vi "Home.vi"(7 "error in (no error)":errorcluster caption="에러 입력(에러 없음)") -> (0 "error out":errorcluster caption="에러 출력", 2 "State":T1)   [LabVIEW 2019]
uses:
  controller/patientListBtn.ctl
  controller/robotBtn.ctl
  controller/alignBtn.ctl
  controller/exitBtn.ctl
  controller/logoutBtn.ctl
  controller/pannelState.ctl
  <vilib>/Utility/miscctls.llb/LVPointTypeDef.ctl
  globalValue.vi
panel:
  out "roleId":string
  in  "Help Button":bool
  in  "LogOut Button":T2
  in  "Exit Button":T3
  out "userNm":string
  in  "Select Button":T4(radio)
  # "|"
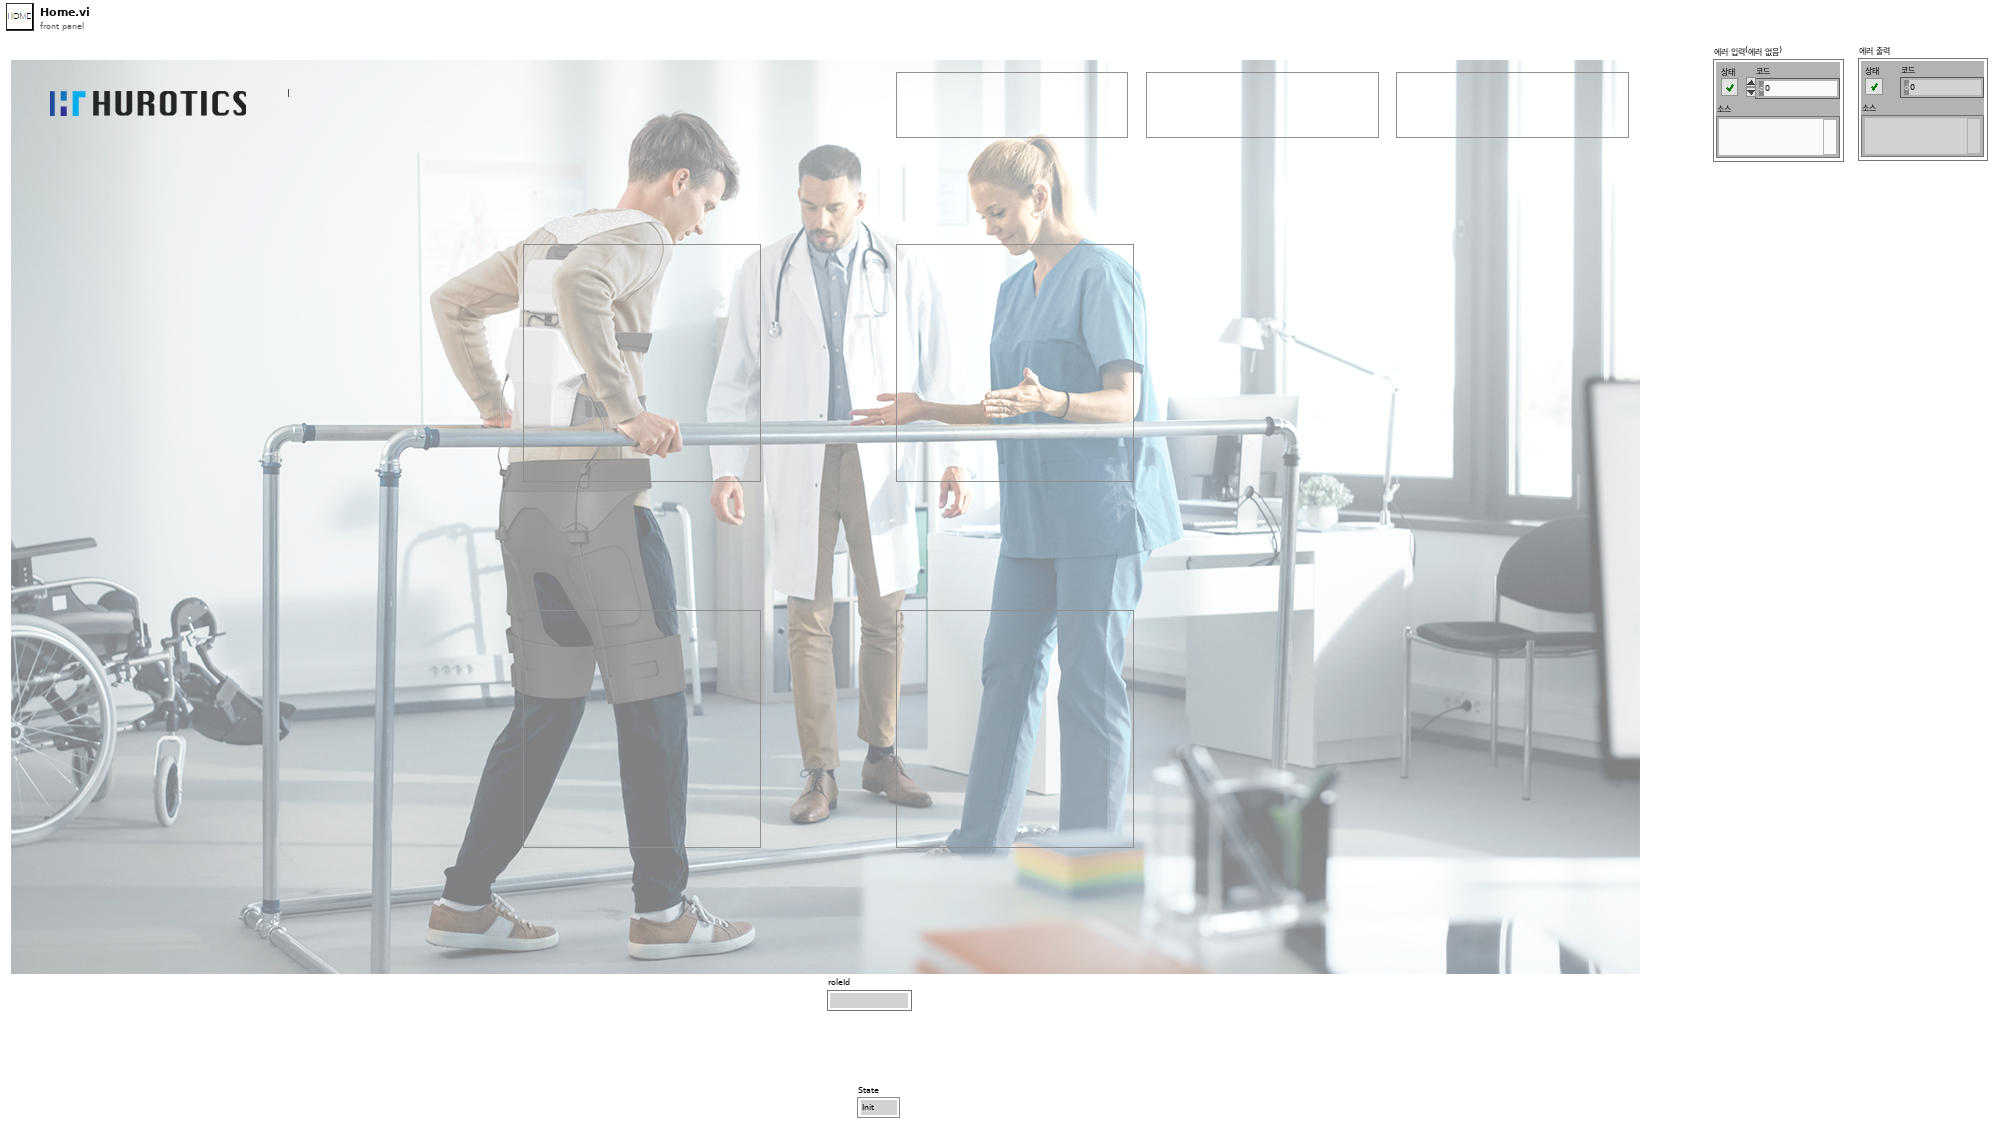
[diagram p1: front panel]
types:
  T1 = typedef "pannelState.ctl" = enum16{"Init", "LogIn", "SignUpView", "Home", "Management_patientList", "Management_patientTrashtList", "Management_patientCreate", "Management_patientUpdate", "Management_patientTraining", "Management_patientTrainingDetail", "H-MEDI PatientList", "H-MEDI HardwareCtl", "Adjust", "FineTuning", "UserList", "UserDetail", "Exit"}
  T2 = typedef "logoutBtn.ctl" = bool
  T3 = typedef "exitBtn.ctl" = bool
  T4 = enum32{"선택 없음", "Select 1", "Select 2", "Select 3", "Select 4"}
  T5 = typedef "LVPointTypeDef.ctl" = cluster{"Horizontal":i16, "Vertical":i16}
  T6 = enum16{"connection", "create", "read", "update", "delete", "close"}
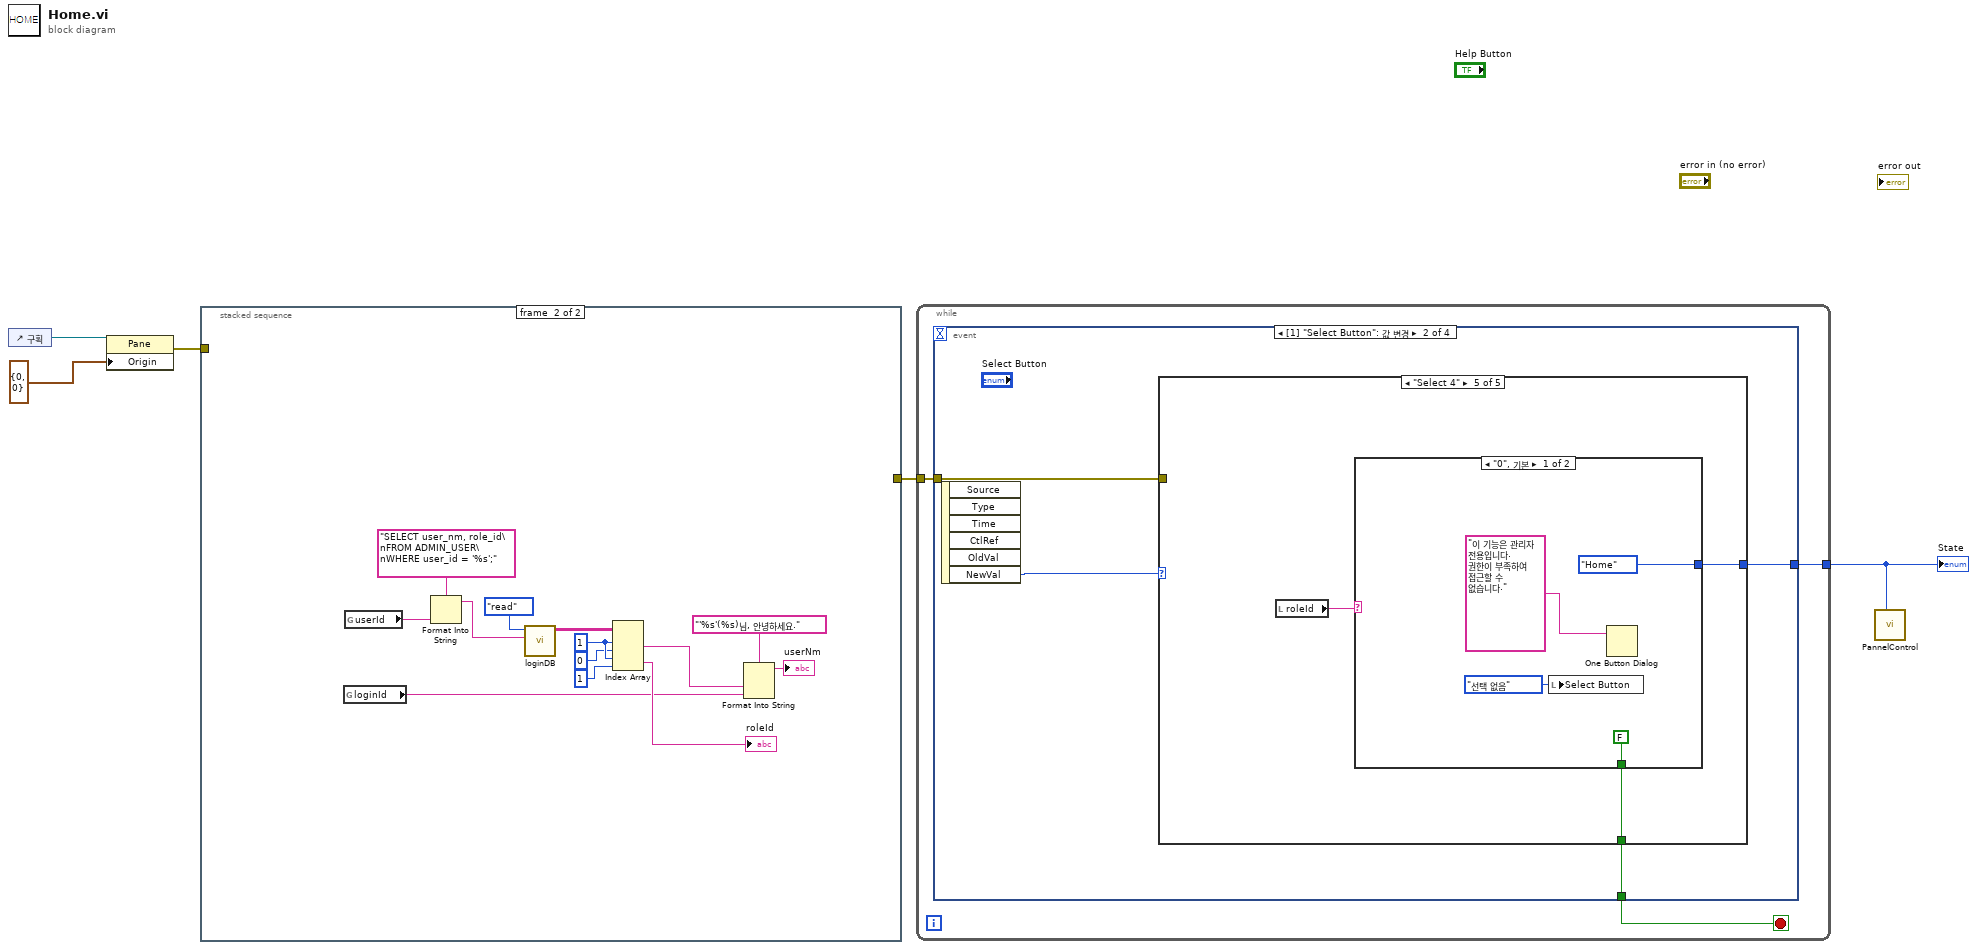
[diagram p0: block diagram]
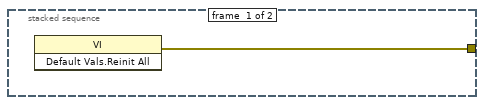
[diagram p2: hidden frame]
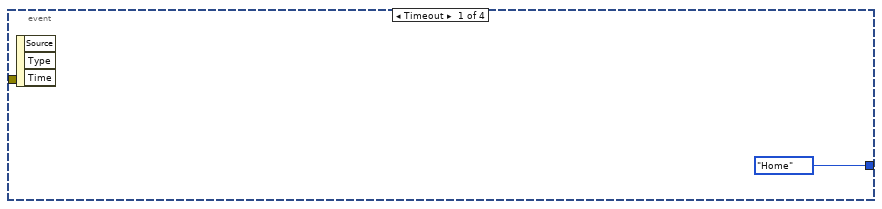
[diagram p3: hidden frame]
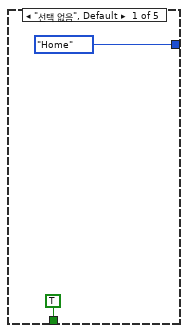
[diagram p4: hidden frame]
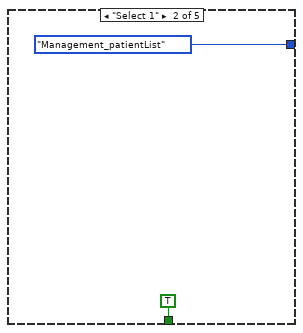
[diagram p5: hidden frame]
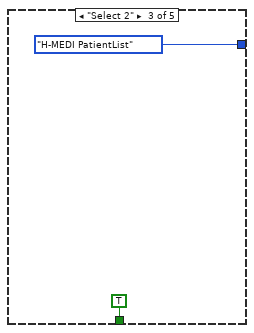
[diagram p6: hidden frame]
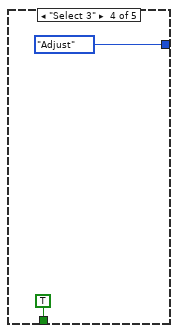
[diagram p7: hidden frame]
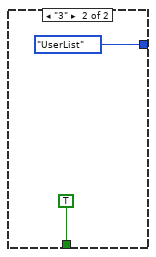
[diagram p8: hidden frame]
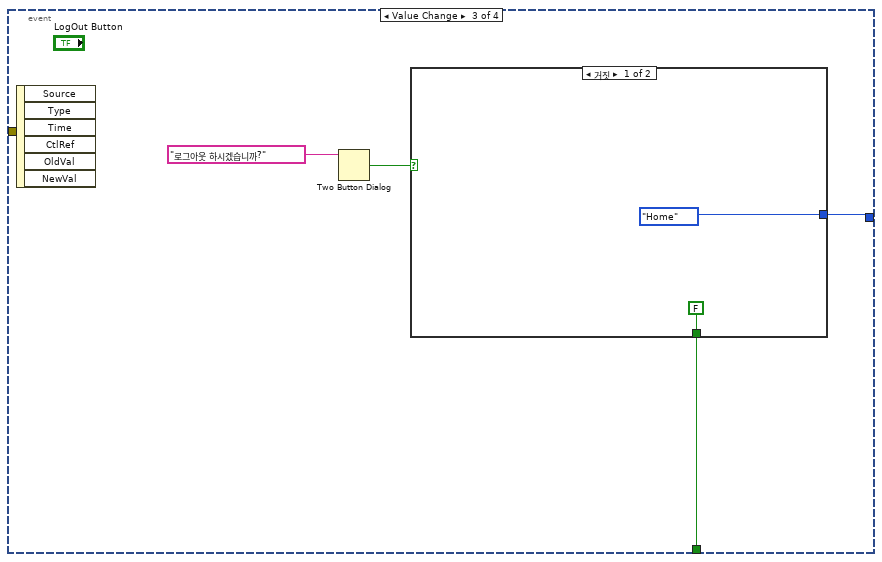
[diagram p9: hidden frame]
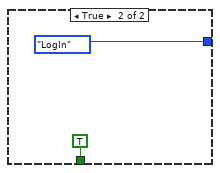
[diagram p10: hidden frame]
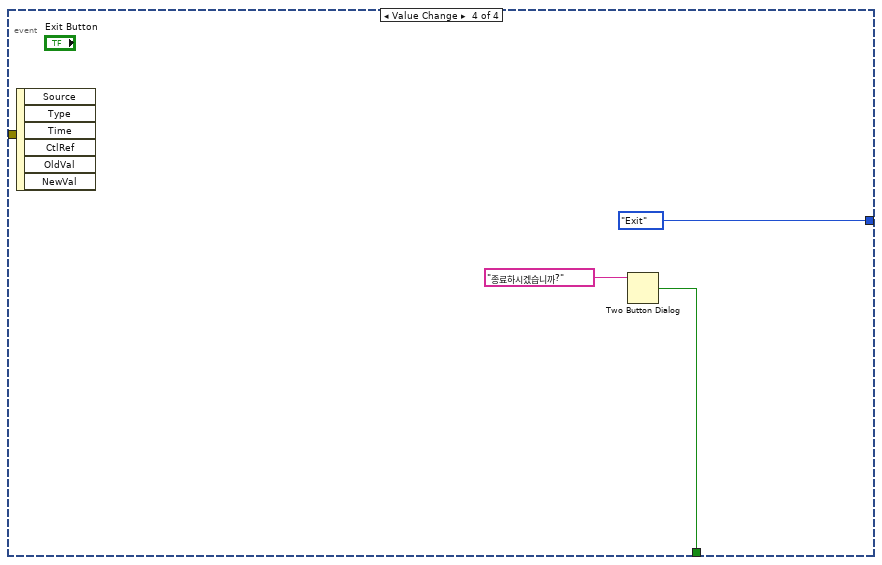
[diagram p11: hidden frame]
diagram:
  n1 = control-ref of="구획"() -> (w3:refnum<vi>)
  n2 = property class="Pane"(reference=w3, "Origin"=T5 {"Horizontal"=0, "Vertical"=0} ("원점")) -> (error out=w2:errorcluster)  [unwired: 1 in, 1 out]
  n3 = stacked-sequence {
    tunnel: [w6 _] -> w5
    tunnel: w2 -> [_ _]
    frame #0 {
      n4 = invoke class="VI" method="Default Vals.Reinit All"() -> (error out=w6:errorcluster)  [unwired: 3 in, 2 out]
    }
    frame #1 {
      w12 = 1 ("인덱스 (행)")
      n5 = global read "globalValue.vi" "loginId"() -> (w7:string)
      n6 = global read "globalValue.vi" "userId"() -> (w14:string)
      n7 = Format Into String(format string="SELECT user_nm, role_id\nFROM ADMIN_USER\nWHERE user_id = '%s';" ("Query"), w14) -> (resulting string=w19:string)  [unwired: 2 in, 1 out]
      n8 = call "loginDB.vi"("Query"=w19, "State"=T6."read") -> ("Result Set"=w18:string[][])  [unwired: 7 in, 1 out]
      n9 = Index Array(array=w18, index (row) #1=w12, index (col) #1=0 ("비활성화된 인덱스 (열)"), index (row) #2=w12, index (col) #2=1 ("비활성화된 인덱스 (열)")) -> (element #1=w16:string, element #2=→"roleId":string)
      n10 = Format Into String(format string="'%s'(%s)님, 안녕하세요." ("포맷 문자열"), w16, w7) -> (resulting string=→"userNm":string)  [unwired: 2 in, 1 out]
    }
  }
  n11 = while {
    tunnel: w5 -> [w21]
    tunnel: [w20] -> w1
    stop <- w22 stop-if-true
    n12 = event shown="[1] \"Select Button\": 값 변경" {
      selector: _ -> [_ _ _ _]
      dyn-events: _ -> [_ _ _ _]
      timeout: _ -> [_ _ _ _]
      tunnel: [_ w24 w45 w53] -> w22
      tunnel: w21 -> [_ w26 _ _]
      tunnel: [pannelState."Home" ("State") w25 w46 pannelState."Exit" ("State")] -> w20
      event Timeout {
        n13 = event-data() -> ()  [unwired: 1 in, 3 out]
      }
      event "Select Button": Value Change {
        n14 = event-data() -> ("NewVal"=w27:T4)  [unwired: 1 in, 5 out]
        n15 = case shown="\"Select 4\"" w27 {
          tunnel: w26 -> [_ _ _ _ _]
          tunnel: [pannelState."Home" ("State") pannelState."Management_patientList" ("State") pannelState."H-MEDI PatientList" ("State") pannelState."Adjust" ("State") w38] -> w25
          tunnel: [TRUE TRUE TRUE TRUE w37] -> w24
          frame "선택 없음", Default {
          }
          frame "Select 1" {
          }
          frame "Select 2" {
          }
          frame "Select 3" {
          }
          frame "Select 4" {
            n16 = local read "roleId"() -> (w36:string)
            n17 = case shown="\"0\", 기본" w36 {
              tunnel: [pannelState."Home" ("State") pannelState."UserList" ("State")] -> w38
              tunnel: [FALSE TRUE] -> w37
              frame "0", Default {
                n18 = local write "Select Button"(T4."선택 없음" ("Select Button")) -> ()
                n19 = One Button Dialog(message="이 기능은 관리자 전용입니다. 권한이 부족하여 접근할 수 없습니다." ("메시지")) -> ()  [unwired: 1 in, 1 out]
              }
              frame "3" {
              }
            }
          }
        }
      }
      event Value Change {
        n20 = event-data() -> ()  [unwired: 1 in, 6 out]
        n21 = Two Button Dialog(message="로그아웃 하시겠습니까?" ("메시지")) -> (T button?=w47:bool)  [unwired: 2 in]
        n22 = case shown="거짓" w47 {
          tunnel: [pannelState."Home" ("State") pannelState."LogIn" ("State")] -> w46
          tunnel: [FALSE TRUE] -> w45
          frame False {
          }
          frame True {
          }
        }
      }
      event Value Change {
        n23 = event-data() -> ()  [unwired: 1 in, 6 out]
        n24 = Two Button Dialog(message="종료하시겠습니까?" ("메시지")) -> (T button?=w53:bool)  [unwired: 2 in]
      }
    }
  }
  "State" <- w1
  n25 = call "PannelControl.vi"("State"=w1) -> ()  [unwired: 10 in, 1 out]
